vi "Open Settings.vi"(8 "error in (no error)":errorcluster, 10 "Schedule":u16, 11 "Properties in":T1) -> (0 "error out":errorcluster, 3 "Properties out":T1)   [LabVIEW 2013]
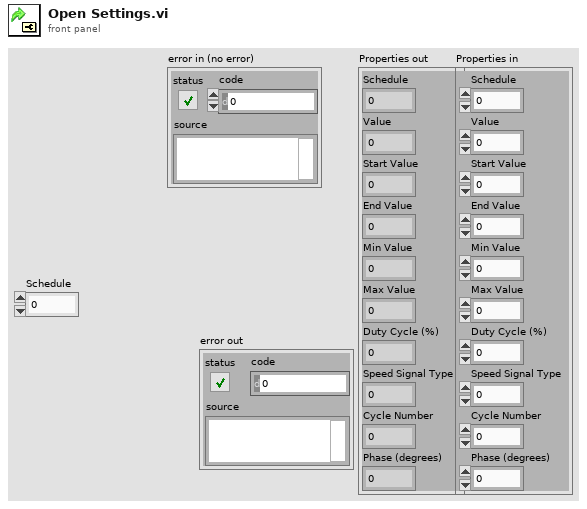
[diagram p1: front panel]
types:
  T1 = cluster{"Schedule":u16, "Value":dbl, "Start Value":dbl, "End Value":dbl, "Min Value":dbl, "Max Value":dbl, "Duty Cycle (%)":dbl, "Speed Signal Type":u16, "Cycle Number":dbl, "Phase (degrees)":dbl}
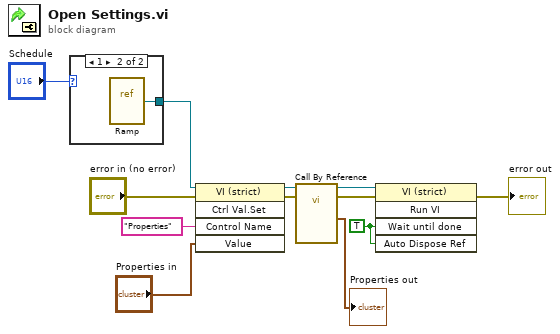
[diagram p0: block diagram]
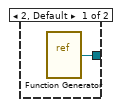
[diagram p2: hidden frame]
diagram:
  w2 = TRUE ("Wait Until Done")
  n1 = case shown="1" "Schedule" {
    tunnel: [w13 w14] -> w9
    frame 2, Default {
      n2 = vi-ref "Function Generator.vi"() -> (w13:refnum<vi>)
    }
    frame 1 {
      n3 = vi-ref "Ramp.vi"() -> (w14:refnum<vi>)
    }
  }
  n4 = invoke class="VI (strict)" method="Ctrl Val.Set"(reference=w9, error in="error in (no error)", "Control Name"="Properties", "Value"="Properties in") -> (reference out=w11:refnum<vi>, error out=w8:errorcluster)  [unwired: 1 in, 3 out]
  n5 = call-by-ref "?"(reference=w11, error in=w8) -> (reference out=w4:refnum<vi>, error out=w3:errorcluster, "Properties"=→"Properties out":T1)  [unwired: 10 in, 1 out]
  n6 = invoke class="VI (strict)" method="Run VI"(reference=w4, error in=w3, "Wait until done"=w2, "Auto Dispose Ref"=w2) -> (error out=→"error out":errorcluster)  [unwired: 1 in, 4 out]
